vi "CANOpen EnableDisable Main Page.vi"(11 "Node Ptr":T1=18446744073709551615 format="%.0x") -> ()   [LabVIEW 2021, in "CANOpen Addon System Explorer.lvlib"]
uses:
  CANOpen Addon System Explorer.lvlib
  <vilib>/NI VeriStand/Custom Device API/Custom Device Item Ref.ctl
  Shared/CANOpen Addon GUID Lookup Global.vi
  <vilib>/NI VeriStand/Custom Device API/Custom Device API.lvlib
  Shared/CANOpen Addon Shared.lvlib
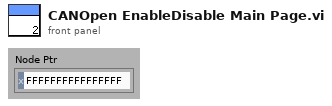
[diagram p1: front panel]
types:
  T1 = typedef "Custom Device API.lvlib/Custom Device Item Ref.ctl" = u64
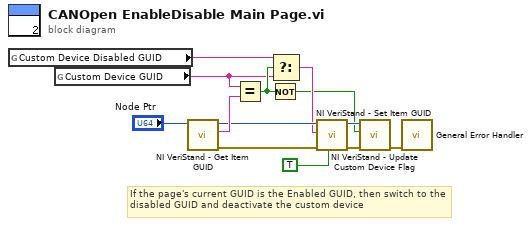
[diagram p0: block diagram]
diagram:
  # "If the page's current GUID is the Enabled GUID, then switch to the disabled GUID and deactivate the custom device"
  n1 = global read "CANOpen Addon GUID Lookup Global.vi" "Custom Device Disabled GUID"() -> (w1:string)
  n2 = global read "CANOpen Addon GUID Lookup Global.vi" "Custom Device GUID"() -> (w2:string)
  n3 = call <vilib>:"NI VeriStand - Get Item GUID.vi"("Item Ref in"="Node Ptr") -> ("error out"=w10:errorcluster, "GUID"=w12:string, "Item Ref out"=w9:T1)  [unwired: 8 in]
  n4 = Equal?(x=w2, y=w12) -> (x = y?=w4:bool)
  n5 = Not(x=w4) -> (.not. x?=w3:bool)
  n6 = Select(t=w1, s=w4, f=w2) -> (s? t:f=w8:string)
  n7 = call <vilib>:"NI VeriStand - Set Item GUID.vi"("Refresh System Explorer Tree? (F)"=TRUE, "error in (no error)"=w10, "GUID"=w8, "Item Ref in"=w9) -> ("error out"=w7:errorcluster, "Item Ref out"=w6:T1)  [unwired: 6 in]
  n8 = call <vilib>:"NI VeriStand - Update Custom Device Flag.vi"("error in (no error)"=w7, "Is Custom Device Active?"=w3, "Device Ref in"=w6) -> ("error out"=w5:errorcluster)  [unwired: 7 in, 1 out]
  n9 = call <vilib>:"General Error Handler.vi"("error in (no error)"=w5) -> ()  [unwired: 10 in, 5 out]
